vi "spilib_write.vi"(8 "error in (no error)":errorcluster, 10 "send_buf":i8[](array[numeric]), 11 "handle":i32) -> (0 "error out":errorcluster, 3 "handle out":i32)   [LabVIEW 2017]
uses:
  <vilib>/Utility/error.llb/Error Cluster From Error Code.vi
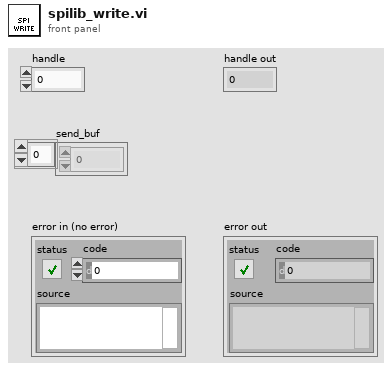
[diagram p1: front panel]
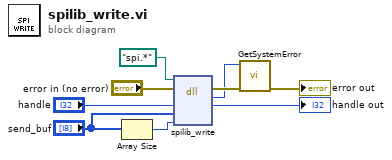
[diagram p0: block diagram]
diagram:
  n1 = Array Size(array="send_buf") -> (size(s)=w2:i32)
  n2 = dll-call lib="?" fn="spilib_write"(path in=path "spi.*", error in="error in (no error)", "handle"="handle", "send_buf"="send_buf", "size"=w2) -> (error out=w8:errorcluster, "return type"=w6:i32, "handle"=→"handle out":i32)  [unwired: 3 in, 1 out]
  n3 = call <vilib>:"GetSystemError.vi"("error in (no error)"=w8, "Retval"=w6) -> ("error out"=→"error out":errorcluster)  [unwired: 9 in]
